vi "GetNoteFrequencies.vi"(11 "# harmonics":i32=40) -> (1 "frequencies":dbl[](array[numeric]), 2 "Table":string[][](table)=[["G3", "196.00", "176.02"], [" G#3/Ab3 ", "207.65", "166.14"], ["A3", "220.00", "156.82"], [" A#3/Bb3 ", "233.08", "148.02"], ["B3", "246.94", "139.71"], ["C4", "261.63", "131.87"], [" C#4/Db4 ", "277.18", "124.47"], ["D4", "293.66", "117.48"], [" D#4/Eb4 ", "311.13", "110.89"], ["E4", "329.63", "104.66"], ["F4", "349.23", "98.79"], [" F#4/Gb4 ", "369.99", "93.24"], ["G4", "392.00", "88.01"], [" G#4/Ab4 ", "415.30", "83.07"], ["A4", "440.00", "78.41"], [" A#4/Bb4 ", "466.16", "74.01"], ["B4", "493.88", "69.85"], ["C5", "523.25", "65.93"], [" C#5/Db5 ", "554.37", "62.23"], ["D5", "587.33", "58.74"], [" D#5/Eb5 ", "622.25", "55.44"], ["E5", "659.25", "52.33"], ["F5", "698.46", "49.39"], [" F#5/Gb5 ", "739.99", "46.62"], ["G5", "783.99", "44.01"], [" G#5/Ab5 ", "830.61", "41.54"], ["A5", "880.00", "39.20"], [" A#5/Bb5 ", "932.33", "37.00"], ["B5", "987.77", "34.93"], ["C6", "1046.50", "32.97"], [" C#6/Db6 ", "1108.73", "31.12"], ["D6", "1174.66", "29.37"], [" D#6/Eb6 ", "1244.51", "27.72"], ["E6", "1318.51", "26.17"], ["F6", "1396.91", "24.70"], [" F#6/Gb6 ", "1479.98", "23.31"], ["G6", "1567.98", "22.00"], [" G#6/Ab6 ", "1661.22", "20.77"], ["A6", "1760.00", "19.60"], [" A#6/Bb6 ", "1864.66", "18.50"], ["B6", "1975.53", "17.46"], ["C7", "2093.00", "16.48"], [" C#7/Db7 ", "2217.46", "15.56"], ["D7", "2349.32", "14.69"], [" D#7/Eb7 ", "2489.02", "13.86"], ["E7", "2637.02", "13.08"], ["F7", "2793.83", "12.35"], [" F#7/Gb7 ", "2959.96", "11.66"], ["G7", "3135.96", "11.00"], [" G#7/Ab7 ", "3322.44", "10.38"], ["A7", "3520.00", "9.80"], ["A#7/Bb7 ", "3729.31", "9.25"], ["B7", "3951.07", "8.73"]], 3 "Labels":T1(array[cluster]))   [LabVIEW 2022 SP3]
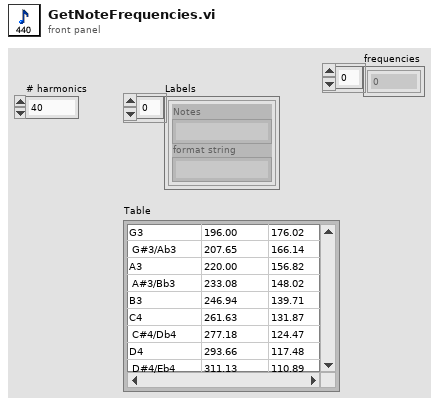
[diagram p1: front panel]
types:
  T1 = cluster{"Notes":string, "format string":string}[]
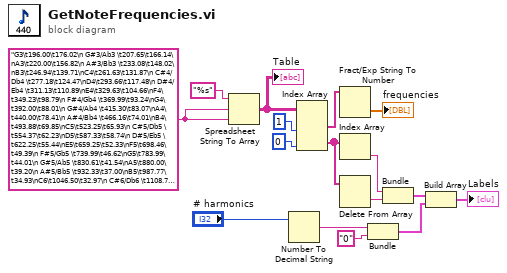
[diagram p0: block diagram]
diagram:
  w15 = "G3\t196.00\t176.02\n G#3/Ab3 \t207.65\t166.14\nA3\t220.00\t156.82\n A#3/Bb3 \t233.08\t148.02\nB3\t246.94\t139.71\nC4\t261.63\t131.87\n C#4/Db4 \t277.18\t124.47\nD4\t293.66\t117.48\n D#4/Eb4 \t311.13\t110.89\nE4\t329.63\t104.66\nF4\t349.23\t98.79\n F#4/Gb4 \t369.99\t93.24\nG4\t392.00\t88.01\n G#4/Ab4 \t415.30\t83.07\nA4\t440.00\t78.41\n A#4/Bb4 \t466.16\t74.01\nB4\t493.88\t69.85\nC5\t523.25\t65.93\n C#5/Db5 \t554.37\t62.23\nD5\t587.33\t58.74\n D#5/Eb5 \t622.25\t55.44\nE5\t659.25\t52.33\nF5\t698.46\t49.39\n F#5/Gb5 \t739.99\t46.62\nG5\t783.99\t44.01\n G#5/Ab5 \t830.61\t41.54\nA5\t880.00\t39.20\n A#5/Bb5 \t932.33\t37.00\nB5\t987.77\t34.93\nC6\t1046.50\t32.97\n C#6/Db6 \t1108.73\t31.12\nD6\t1174.66\t29.37\n D#6/Eb6 \t1244.51\t27.72\nE6\t1318.51\t26.17\nF6\t1396.91\t24.70\n F#6/Gb6 \t1479.98\t23.31\nG6\t1567.98\t22.00\n G#6/Ab6 \t1661.22\t20.77\nA6\t1760.00\t19.60\n A#6/Bb6 \t1864.66\t18.50\nB6\t1975.53\t17.46\nC7\t2093.00\t16.48\n C#7/Db7 \t2217.46\t15.56\nD7\t2349.32\t14.69\n D#7/Eb7 \t2489.02\t13.86\nE7\t2637.02\t13.08\nF7\t2793.83\t12.35\n F#7/Gb7 \t2959.96\t11.66\nG7\t3135.96\t11.00\n G#7/Ab7 \t3322.44\t10.38\nA7\t3520.00\t9.80\nA#7/Bb7 \t3729.31\t9.25\nB7\t3951.07\t8.73\nC8\t4186.01\t8.24\n C#8/Db8 \t4434.92\t7.78\nD8\t4698.63\t7.34\n D#8/Eb8 \t4978.03\t6.93\nE8\t5274.04\t6.54\nF8\t5587.65\t6.17\n F#8/Gb8 \t5919.91\t5.83\nG8\t6271.93\t5.50\n G#8/Ab8 \t6644.88\t5.19\nA8\t7040.00\t4.90\n A#8/Bb8 \t7458.62\t4.63\nB8\t7902.13\t4.37" ("Notes")
  n1 = Spreadsheet String To Array(format string="%s", spreadsheet string=w15, array type (2D Dbl)=w15) -> (array=w3:string[][])  [unwired: 1 in]
  "Table" <- w3
  n2 = Number To Decimal String(number="# harmonics") -> (decimal integer string=w11:string)  [unwired: 1 in]
  n3 = Index Array(array=w3, index (col) #1=1 ("disabled index (col)"), index (col) #2=0 ("disabled index (col)")) -> (element #1=w14:string[], element #2=w6:string[])  [unwired: 2 in]
  n4 = Fract/Exp String To Number(string=w14) -> (number=→"frequencies":dbl[])  [unwired: 3 in, 1 out]
  n5 = Index Array(array=w6) -> (element=w7:string)  [unwired: 1 in]
  n6 = Delete From Array(array=w6) -> (deleted portion=w8:string)  [unwired: 2 in, 1 out]
  n7 = Bundle(w11, "format string"="0") -> (w10:cluster{string, "format string":string})  [unwired: 1 in]
  n8 = Bundle("Notes"=w7, "Notes"=w8) -> (w9:cluster{"Notes":string, "Notes":string})  [unwired: 1 in]
  n9 = Build Array(w9, w10) -> (→"Labels":T1)
